vi "create_LSID.vi"(8 "error in (no error)":errorcluster, 11 "GenericPlugin in":refnum<class "GenericComponent.lvclass">) -> (0 "error out":errorcluster, 2 "current LSID":T1, 3 "GenericPlugin out":refnum<class "GenericComponent.lvclass">)   [LabVIEW 2010, in "GenericComponent.lvclass"]
uses:
  GenericComponent.lvclass
  clusters/LSID_cluster.ctl
  GenericComponent.lvclass/GenericComponent.ctl
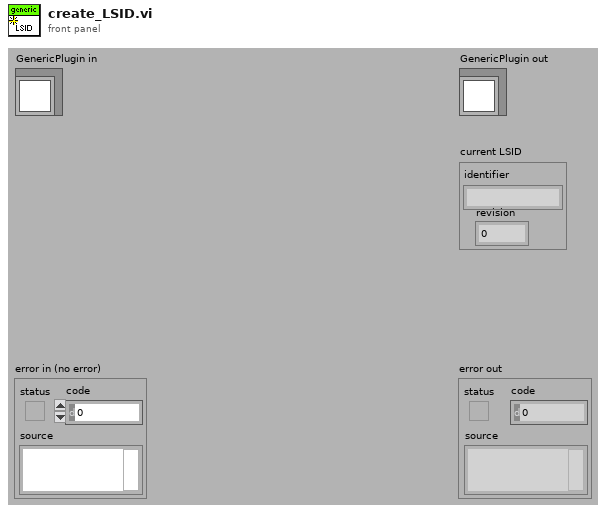
[diagram p1: front panel]
types:
  T1 = typedef "LSID_cluster.ctl" = cluster{"identifier":string, "revision":i32}
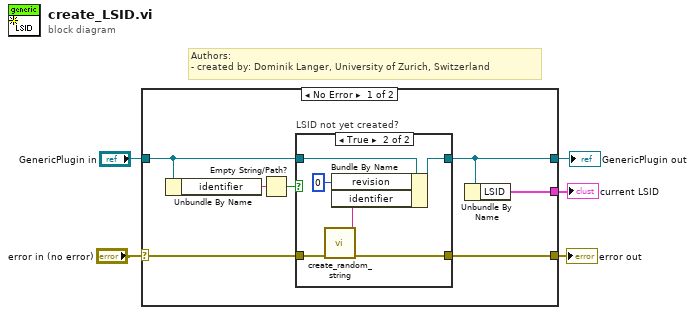
[diagram p0: block diagram]
diagram:
  # "Authors: \n- created by: Dominik Langer, University of Zurich, Switzerland"
  n1 = case shown="No Error" "error in (no error)" {
    selector: "error in (no error)" -> [w11 w22]
    tunnel: [w9 w22] -> w4
    tunnel: [w7 w21] -> w2
    tunnel: "GenericPlugin in" -> [w10 w21]
    tunnel: [w6 _] -> w1
    frame No Error {
      n2 = Unbundle By Name(w10) -> ("identifier"=w12:string)
      n3 = Empty String/Path?(string/path=w12) -> (empty?=w8:bool)
      n4 = case "LSID not yet created?" shown="True" w8 {
        tunnel: w11 -> [w13 w20]
        tunnel: w10 -> [w14 w16]
        tunnel: [w14 w15] -> w7
        tunnel: [w13 w17] -> w9
        frame False {
        }
        frame True {
          n5 = call "create_random_string.vi"("error in (no error)"=w20) -> ("error out"=w17:errorcluster, "random string"=w19:string)  [unwired: 9 in]
          n6 = Bundle By Name(cluster=w16, "revision"=0 ("LSID.revision"), "identifier"=w19) -> (w15:refnum<class "GenericComponent.lvclass">)
        }
      }
      n7 = Unbundle By Name(w7) -> ("LSID"=w6:T1)
    }
    frame Error {
    }
  }
  "error out" <- w4
  "GenericPlugin out" <- w2
  "current LSID" <- w1
